vi "Conf External Instrument.vi"(4 "Channel Advance Source \n(0:External)":enum16{"External", "Bus", "Immediate"}(ring), 5 "Check Parameter (0:CH Adv Src)":T1(ring), 6 "Channel List (empty)":string, 7 "Set/Check (F:Set)":bool, 8 "error in (no error)":errorcluster, 9 "Internal DMM? (F:Off)":bool, 10 "4-wire Scanning (F:Off)":bool, 11 "VISA Resource Name":refnum<visa-resource-name>) -> (0 "error out":errorcluster, 2 "Configuration?":string, 3 "VISA Resource Name Out":refnum<visa-resource-name>)   [LabVIEW 2016, in "Agilent 34970.lvlib"]
doc: "This VI allows you to configure the instrument for scanning with an external DMM."
uses:
  Agilent 34970.lvlib
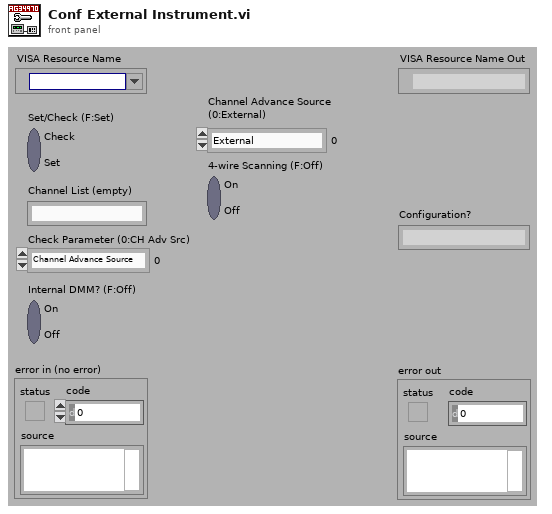
[diagram p1: front panel]
types:
  T1 = enum16{"Channel Advance Source", "4-wire State?", "Internal DMM State"}
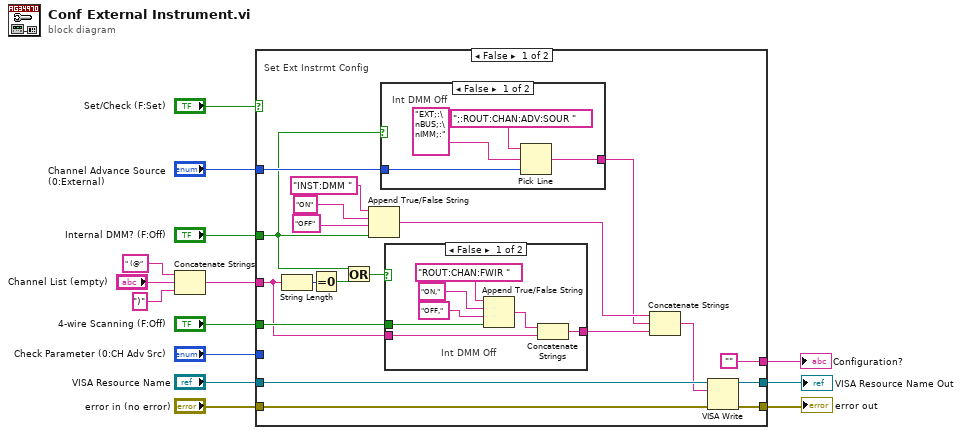
[diagram p0: block diagram]
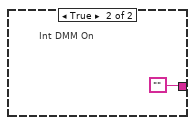
[diagram p2: hidden frame]
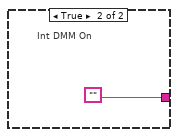
[diagram p3: hidden frame]
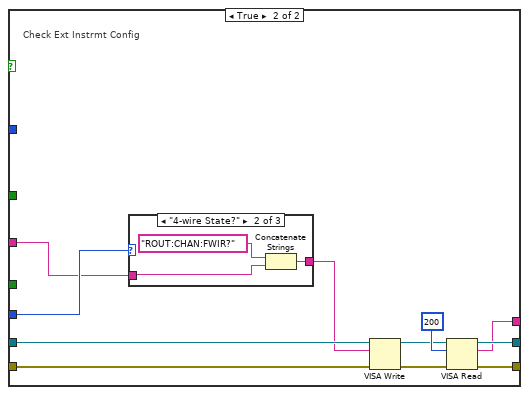
[diagram p4: hidden frame]
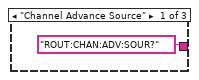
[diagram p5: hidden frame]
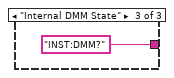
[diagram p6: hidden frame]
diagram:
  n1 = Concatenate Strings(" (@", "Channel List (empty)", ")") -> (w7:string)
  n2 = case shown="False" "Set/Check (F:Set)" {
    tunnel: "Channel Advance Source \n(0:External)" -> [w33 _]
    tunnel: "4-wire Scanning (F:Off)" -> [w32 _]
    tunnel: "Internal DMM? (F:Off)" -> [w16 _]
    tunnel: w7 -> [w22 w49]
    tunnel: "VISA Resource Name" -> [w29 w52]
    tunnel: "error in (no error)" -> [w28 w51]
    tunnel: [w25 w54] -> w4
    tunnel: [w24 w53] -> w3
    tunnel: ["" w48] -> w6
    tunnel: "Check Parameter (0:CH Adv Src)" -> [_ w50]
    frame False {
      # "Set Ext Instrmt Config"
      n3 = String Length(string=w22) -> (length=w23:i32)
      n4 = Equal To 0?(x=w23) -> (x = 0?=w15:bool)
      n5 = Or(x=w16, y=w15) -> (x .or. y?=w17:bool)
      n6 = Append True/False String(1:w16, 2:"OFF" ("multi-line string"), 3:"ON" ("multi-line string"), 4:"INST:DMM ") -> (0:w20:string)
      n7 = case shown="False" w16 {
        tunnel: [w37 ""] -> w19
        tunnel: w33 -> [w36 _]
        frame False {
          # "Int DMM Off"
          n8 = Pick Line(string ("")=";:ROUT:CHAN:ADV:SOUR ", multi-line string="EXT;:\nBUS;:\nIMM;:", line index=w36) -> (output string=w37:string)
        }
        frame True {
          # "Int DMM On"
        }
      }
      n9 = case shown="False" w17 {
        tunnel: w22 -> [w45 _]
        tunnel: w32 -> [w42 _]
        tunnel: [w39 ""] -> w21
        frame False {
          # "Int DMM Off"
          n10 = Append True/False String(1:w42, 2:"OFF," ("multi-line string"), 3:"ON," ("multi-line string"), 4:"ROUT:CHAN:FWIR ") -> (0:w44:string)
          n11 = Concatenate Strings(w44, w45) -> (w39:string)
        }
        frame True {
          # "Int DMM On"
        }
      }
      n12 = Concatenate Strings(w20, w19, w21) -> (w27:string)
      n13 = VISA Write(VISA resource name=w29, write buffer=w27, error in (no error)=w28) -> (VISA resource name out=w25:refnum<visa-resource-name>, error out=w24:errorcluster)  [unwired: 1 out]
    }
    frame True {
      # "Check Ext Instrmt Config"
      n14 = case shown="\"4-wire State?\"" w50 {
        tunnel: w49 -> [_ w60 _]
        tunnel: ["ROUT:CHAN:ADV:SOUR?" w59 "INST:DMM?"] -> w47
        frame "Channel Advance Source" {
        }
        frame "4-wire State?" {
          n15 = Concatenate Strings("ROUT:CHAN:FWIR?", w60) -> (w59:string)
        }
        frame "Internal DMM State" {
        }
      }
      n16 = VISA Write(VISA resource name=w52, write buffer=w47, error in (no error)=w51) -> (VISA resource name out=w56:refnum<visa-resource-name>, error out=w55:errorcluster)  [unwired: 1 out]
      n17 = VISA Read(VISA resource name=w56, byte count=u32 200 ("byte count (0)"), error in (no error)=w55) -> (VISA resource name out=w54:refnum<visa-resource-name>, read buffer=w48:string, error out=w53:errorcluster)  [unwired: 1 out]
    }
  }
  "Configuration?" <- w6
  "error out" <- w3
  "VISA Resource Name Out" <- w4
